vi "sbRIO9632_RT_main_DAC_DC.vi"() -> ()   [LabVIEW 2013]
uses:
  <vilib>/userdefined/High Color/nirio_resource_hc.ctl
  <vilib>/Platform/TimedLoop/XDataNode/timing_clust.ctl
  <vilib>/Platform/TimedLoop/XDataNode/nitl_modes.ctl
  <vilib>/Platform/TimedLoop/XDataNode/wakeup.ctl
  <vilib>/FPGAPlugInAG/sbRIO-9612/niLvFpga_Open_sbRIO-9612.vi
  <vilib>/FPGAPlugInAG/sbRIO-9612/niLvFpga_Run_sbRIO-9612.vi
  <vilib>/Utility/error.llb/Error Cluster From Error Code.vi
  <vilib>/rvi/errors/niLvFpgaAdjustHostInterfaceError.vi
  <vilib>/FPGAPlugInAG/sbRIO-9612/niLvFpga_Close_sbRIO-9612.vi
  <vilib>/platform/TimedLoop/XDataNode/XDataNode.xnode
  <vilib>/rvi/interface/nirviOpenFPGA/nirviOpenFPGA.xnode
  FPGA Bitfiles/sbRIO9612_LTC2642_~87_FPGA Target_sbRIO9632_FPGA_mai~3C.lvbit
  <vilib>/rvi/interface/nirviMethod/nirviMethod.xnode
  <vilib>/rvi/interface/nirviReadWriteControl/nirviReadWriteControl.xnode
  <vilib>/rvi/interface/nirviCloseFPGA/nirviCloseFPGA.xnode
  <vilib>/Platform/TimedLoop/XDataNode/XDNodeRunTimeDep.lvlib
  NiFpgaLv.dll
panel:
  out "error out":errorcluster
  in  "Stop":bool
  out "Pattern":bool[](array[boolean])=[TRUE, FALSE, TRUE, FALSE, TRUE, TRUE, FALSE, FALSE, TRUE, TRUE, TRUE, TRUE, FALSE, FALSE, FALSE, FALSE, TRUE, TRUE, TRUE, TRUE, TRUE, TRUE, TRUE, TRUE, FALSE, FALSE, FALSE, FALSE, FALSE, FALSE, FALSE, TRUE]
  in  "Panel number":u8 max=9 step=1 format="%_1f"
  in  "Channel number":u8(ring)=128 items=["0"=128, "1"=64, "2"=32, "3"=16, "4"=8, "5"=4, "6"=2, "7"=1]
  in  "Dac value":u16=32769 format="%#_6f"
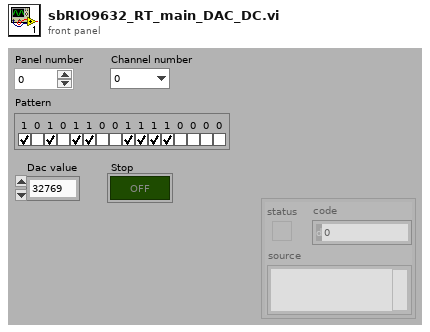
[diagram p1: front panel]
types:
  T1 = typedef "nirio_resource_hc.ctl" = tag
  T2 = typedef "XDNodeRunTimeDep.lvlib/timing_clust.ctl" = cluster{"Expected End [f-1]":u64, "Actual End [f-1]":u64, "Finished Late? [f-1]":bool, "Expected End [i-1]":u64, "Actual End [i-1]":u64, "Finished Late? [i-1]":bool, "Expected Start [i]":u64, "Actual Start [i]":u64, "Expected Start [f]":u64, "Actual Start [f]":u64, "Source Name":string, "Structure Name":string, "Period":i64, "Deadline":i64, "Offset":i64, "Start":i64, "Priority":i32, "Timeout":i32, "Mode":T3, "Wakeup Reason":T4, "Error":errorcluster, "Source Type":string, "Secondary Source Type":string, "Global End Time":u64, "Global Start Time":u64, "Frame Duration":u64, "Iteration Duration":u64, "Assigned CPU":i32, "I/O Scan Engine Mode":u32}
  T3 = typedef "XDNodeRunTimeDep.lvlib/nitl_modes.ctl" = enum32{"No Change", "Process missed periods, maintain original phase", "Discard missed periods, maintain original phase", "Process missed periods, ignore original phase", "Discard missed periods, ignore original phase"}
  T4 = typedef "XDNodeRunTimeDep.lvlib/wakeup.ctl" = enum32{"Normal", "Aborted", "Asynchronous wakeup", "Timing source error", "Timed loop error", "Timeout"}
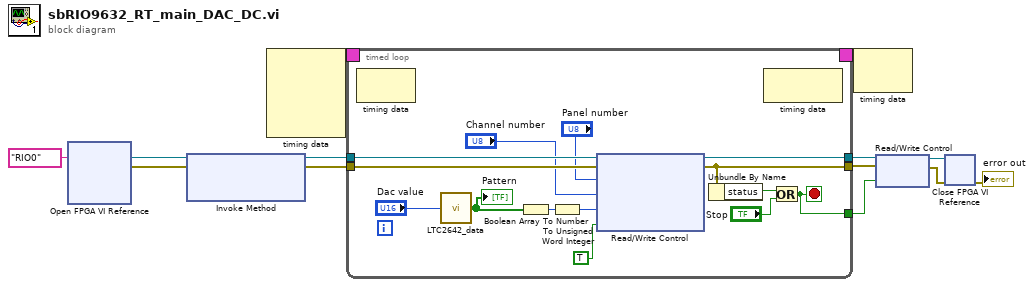
[diagram p0: block diagram]
diagram:
  n1 = xnode "Open FPGA VI Reference"("resource name"=T1 "RIO0") -> ("FPGA VI Reference Out"=w4:refnum<k20>, "error out"=w3:errorcluster)  [unwired: 1 in]
  n2 = xnode "Invoke Method"("FPGA VI Reference In"=w4) -> ("FPGA VI Reference Out"=w1:refnum<k20>)  [unwired: 2 in, 1 out]
  n3 = node-c288() -> (w12:T2)  [unwired: 4 out]
  n4 = timed-loop {
    timing: w12 -> [_]
    timing-out: [_] -> w11
    tunnel: w1 -> [w26]
    tunnel: w3 -> [w25]
    tunnel: [w24] -> w2
    tunnel: [w23] -> w10
    tunnel: [w20] -> w5
    stop <- w20 stop-if-true
    n5 = node-c288() -> ()  [unwired: 2 out]
    n6 = call "LTC2642_data.vi"("Dac value"="Dac value") -> ("Boardi_Data_Pt"=w13:bool[])
    "Pattern" <- w13
    n7 = Boolean Array To Number(Boolean array=w13) -> (number=w19:u32)
    n8 = To Unsigned Word Integer(number=w19) -> (unsigned 16bit integer=w15:u16)
    n9 = xnode "Read/Write Control"("FPGA VI Reference In"=w26, "error in"=w25, "Panel number"="Panel number", "Channel number"="Channel number", "Data"=w15, "Generate"=TRUE) -> ("FPGA VI Reference Out"=w24:refnum<k20>, "error out"=w23:errorcluster)
    n10 = Unbundle By Name(w23) -> ("status"=w22:bool)
    n11 = node-c288() -> ()  [unwired: 2 out]
    n12 = Or(x=w22, y="Stop") -> (x .or. y?=w20:bool)
  }
  n13 = node-c288(w11) -> ()  [unwired: 1 out]
  n14 = xnode "Read/Write Control"("FPGA VI Reference In"=w2, "error in"=w10, "Stop"=w5) -> ("FPGA VI Reference Out"=w9:refnum<k20>, "error out"=w8:errorcluster)
  n15 = xnode "Close FPGA VI Reference"("FPGA VI Reference In"=w9, "error in"=w8) -> ("error out"=→"error out":errorcluster)
